vi "h.DETECTION.SetChannelDetectionSettingId.vi"(8 "error in":errorcluster, 9 "Detection Setting ID":u8, 10 "Channel Number":u8=1 min=1 max=16, 11 "Connection ID":refnum<k5>) -> (0 "error out":errorcluster, 3 "Connection ID out":refnum<k5>)   [LabVIEW 2016, in "h.Library.lvlib"]
uses:
  h.Library.lvlib
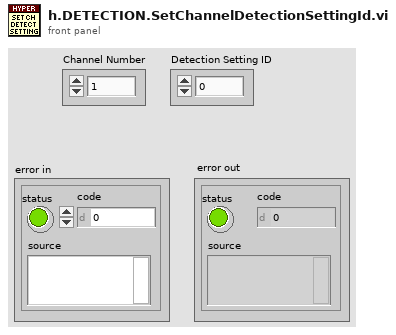
[diagram p1: front panel]
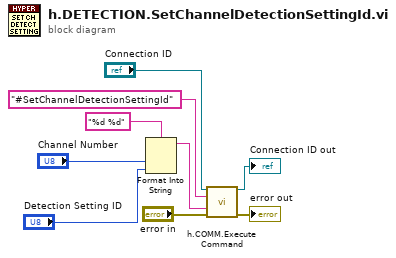
[diagram p0: block diagram]
diagram:
  n1 = Format Into String(format string="%d %d", "Channel Number", "Detection Setting ID") -> (resulting string=w1:string)  [unwired: 2 in, 1 out]
  n2 = call "h.COMM.Execute Command.vi"("Connection ID"="Connection ID", "Command"="#SetChannelDetectionSettingId", "Argument"=w1, "error in"="error in") -> ("Connection ID out"=→"Connection ID out":refnum<k5>, "error out"=→"error out":errorcluster)  [unwired: 4 in, 6 out]
